vi "Byte to Half-Bytes.vi"(9 "Byte In":u8=127 format="%b") -> (2 "Lower Half-byte":u8 format="%b", 3 "Upper Half-Byte":u8 format="%b")   [LabVIEW 2020, in "wamplv.lvlib" / "RawSocket TCP Handler.lvclass"]
uses:
  RawSocket TCP Handler.lvclass
  RawSocket TCP Handler.lvclass/RawSocket TCP Handler.ctl
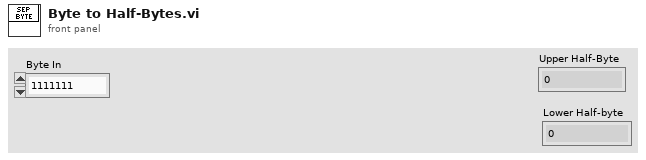
[diagram p1: front panel]
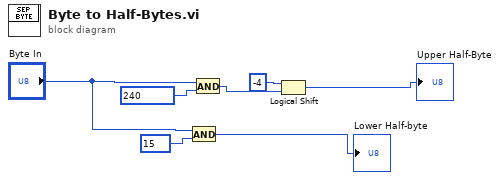
[diagram p0: block diagram]
diagram:
  n1 = And(x="Byte In", y=u8 15) -> (x .and. y?=→"Lower Half-byte":u8)
  n2 = And(x="Byte In", y=u8 240) -> (x .and. y?=w4:u8)
  n3 = Logical Shift(y=i16 -4, x=w4) -> (x << y=→"Upper Half-Byte":u8)
